vi "ReadNew.vi"(0 "object in":refnum<class "CoriFlowBFS1Plus.lvclass">, 5 "error in (no error)":errorcluster) -> (14 "object out":refnum<class "CoriFlowBFS1Plus.lvclass">, 16 "New Data":T1, 19 "error out":errorcluster)   [LabVIEW 2021, in "CoriFlowBFS1Plus.lvclass"]
uses:
  CoriFlowBFS1Plus.lvclass
  CoriFlowBFS1Plus.lvclass/CoriFlowBFS1Plus.ctl
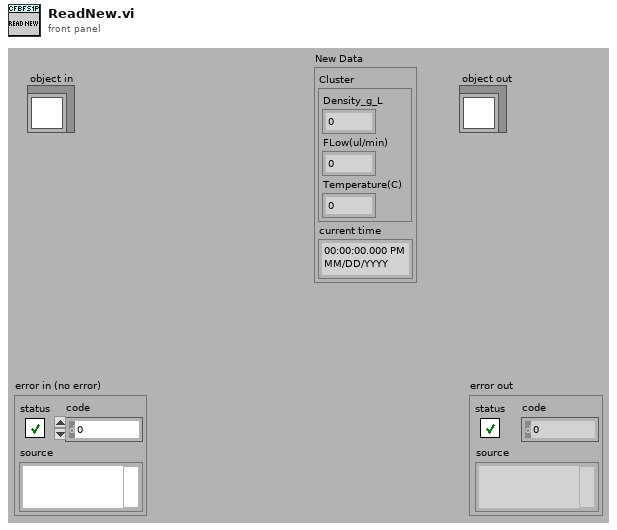
[diagram p1: front panel]
types:
  T1 = cluster{"Cluster":cluster{"Density_g_L":sgl, "FLow(ul/min)":sgl, "Temperature(C)":sgl}, "current time":timestamp}
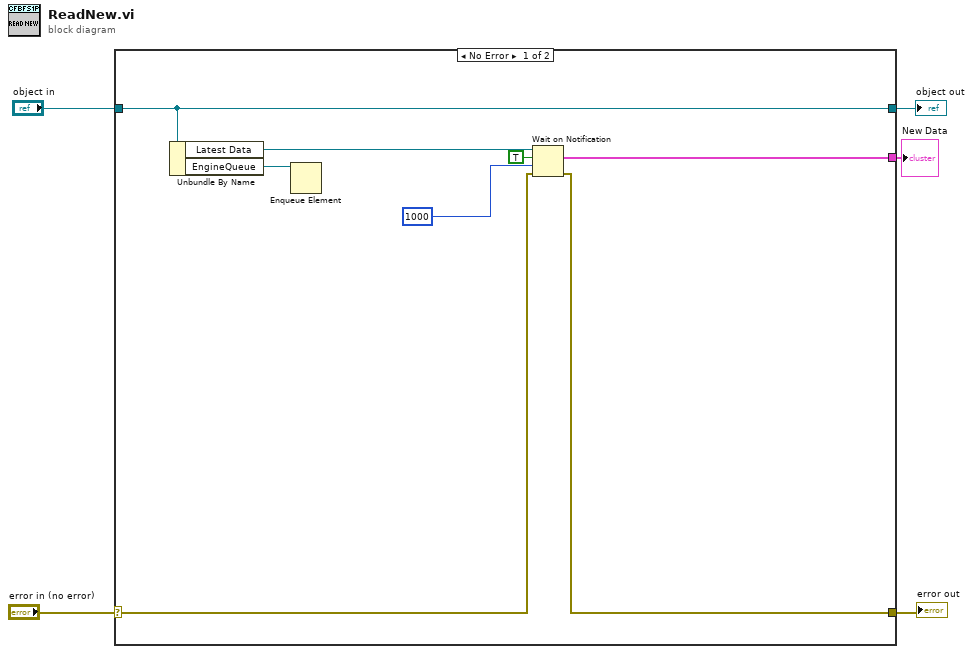
[diagram p0: block diagram]
diagram:
  n1 = case shown="No Error" "error in (no error)" {
    selector: "error in (no error)" -> [w8 w15]
    tunnel: [w7 w15] -> w4
    tunnel: [w13 w14] -> w2
    tunnel: "object in" -> [w13 w14]
    tunnel: [w11 _] -> w1
    frame No Error {
      n2 = Unbundle By Name(w13) -> ("Latest Data"=w12:refnum<notifier>, "EngineQueue"=w6:refnum<queue>)
      n3 = Enqueue Element(queue=w6) -> ()  [unwired: 3 in, 3 out]
      n4 = Wait on Notification(notifier=w12, ignore previous (F)=TRUE, timeout in ms (-1)=1000, error in (no error)=w8) -> (notification=w11:T1, error out=w7:errorcluster)  [unwired: 2 out]
    }
    frame Error {
    }
  }
  "error out" <- w4
  "object out" <- w2
  "New Data" <- w1
